vi "Simple Grab.vi"() -> ()   [LabVIEW 2014]
uses:
  <userlib>/CurtinCode/SimpleViewctrl/SimpleView.xctl
  <userlib>/CurtinCode/Devicectrl/Audio Channel.xctl
panel:
  in  "Audio Channel":T3(xcontrol)
  out "SimpleView 2":T4[](xcontrol)
  in  "Trigger":dbl(slide)=0.04205607476635514 scale=0.0..0.5
  out "SimpleView":T4[](xcontrol)
  in  "stop":bool
  # "Need to change\n\n1. save Device name not device #\n2. reduce Device XCtrl down to device - but with checking\n3. have a setup btn - that lets you control the .ini file - that contains\n     sampling rate\n     channel names\n     etc\n4. autolabel lines on plot - and only show as many as you have lines"
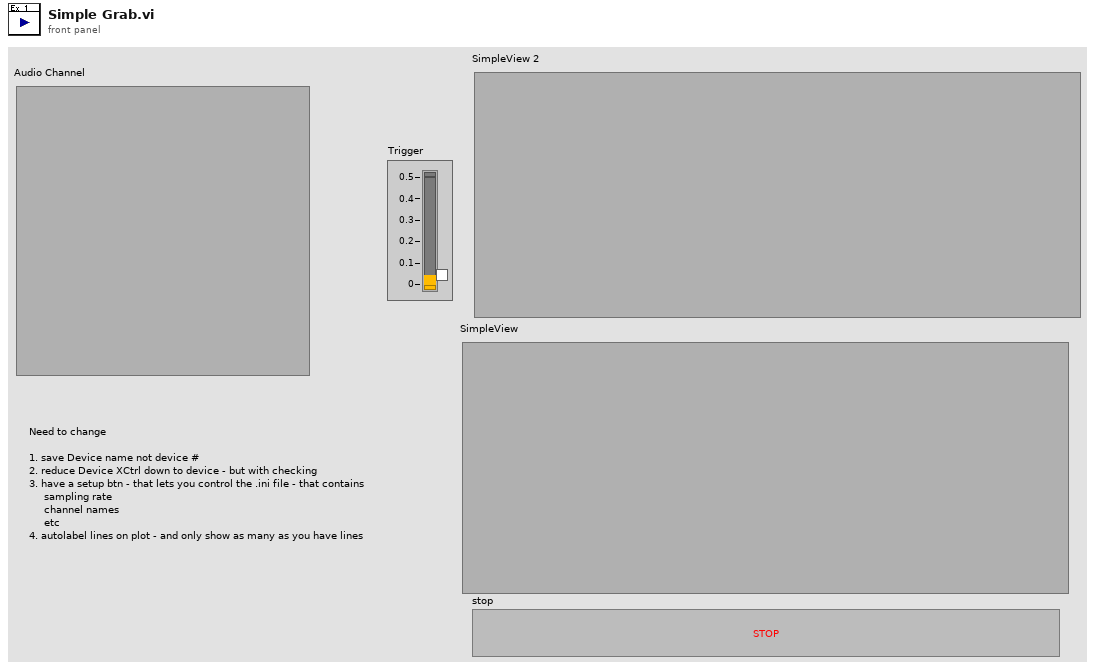
[diagram p1: front panel]
types:
  T1 = typedef "Sampling Mode.ctl" = i32
  T2 = typedef "Sound Data Format.ctl" = cluster{"sample rate (S/s)":dbl, "number of channels":i32, "bits per sample":i32}
  T3 = cluster{"device ID":u32, "Device Name":string, "number of samples/ch":i32, "sample mode":T1, "sound format":T2, "Sample length (sec)":dbl, "Pre-trigger (sec)":dbl}
  T4 = typedef "DataControl.ctl" = cluster{"Settings":T5, "Data":cluster{i32, dbl, "data":dbl[]}[], "Plot type":enum16{"Linear", "log"}}
  T5 = typedef "SettingsControl.ctl" = cluster{"Data Path":path, "Time":timestamp, "Sampling Rate (Hz)":u16, "Device":u16, "pre-trigger (sec)":dbl, "length of sample (sec)":dbl, "trigger value (V)":dbl, "Labels":string[], "Cutoffs (sec)":dbl[], "Freq Bands":dbl[]}
  T6 = typedef "AllDataCtrl.ctl" = cluster{"Data Set":T4, "number of samples/ch":i32, "task ID":T7, "error out":errorcluster, "DAQmx task":refnum<k21>}
  T7 = typedef "Sound Input Task ID.ctl" = u32
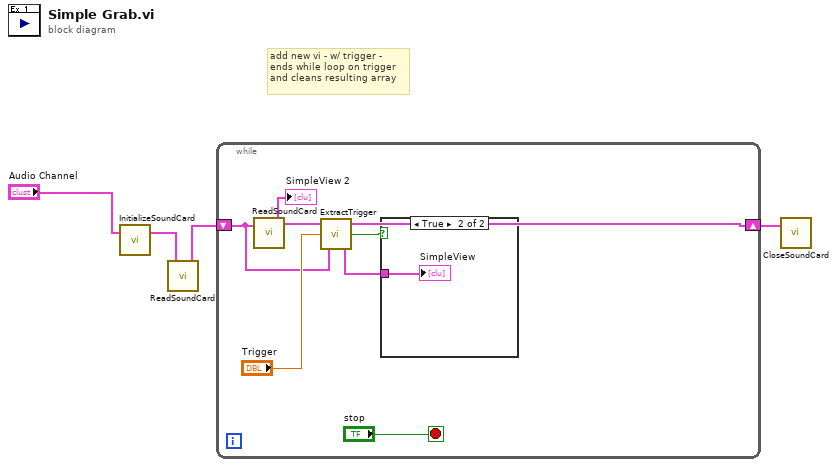
[diagram p0: block diagram]
diagram:
  # "add new vi - w/ trigger - \nends while loop on trigger\nand cleans resulting array"
  n1 = call <userlib>:"InitializeSoundCard.vi"("DeviceXControl"="Audio Channel") -> ("All Info"=w2:T6)  [unwired: 2 in]
  n2 = call <userlib>:"ReadSoundCard.vi"("All Info"=w2) -> ("All Info"=w1:T6)  [unwired: 1 in, 1 out]
  n3 = while {
    shift-right: [w8] -> w4
    shift-left: w1 -> [w10]
    stop <- "stop" stop-if-true
    n4 = call <userlib>:"ReadSoundCard.vi"("All Info"=w10) -> ("Data Set"=→"SimpleView 2":T4[], "All Info"=w9:T6)  [unwired: 1 in]
    n5 = call <userlib>:"ExtractTrigger.vi"(3:"All Info"=w10, "Trigger"="Trigger", 5:"All Info"=w9) -> ("Data Set"=w6:T4[], "Trigger?"=w7:bool, "All Info"=w8:T6)
    n6 = case shown="True" w7 {
      tunnel: w6 -> [_ w13]
      frame False {
      }
      frame True {
        "SimpleView" <- w13
      }
    }
  }
  n7 = call <userlib>:"CloseSoundCard.vi"("All Info"=w4) -> ()  [unwired: 3 in]
